vi "BiFuncHelp_MatrixMult.vi"(9 "B":T1, 10 "A":T1, 11 "Variant":variant) -> (0 "Error":bool, 3 "Output":T1)   [LabVIEW 2019, in "Trajectory_Library.lvlib"]
uses:
  Trajectory_Library.lvlib
  <vilib>/Analysis/Matrix/Datatypes/RealMatrix.ctl
  <vilib>/Analysis/baseanly.llb/Real A x B.vi
  <vilib>/Analysis/NI_AALBase.lvlib
  <vilib>/Analysis/Matrix/NI_Matrix.lvlib
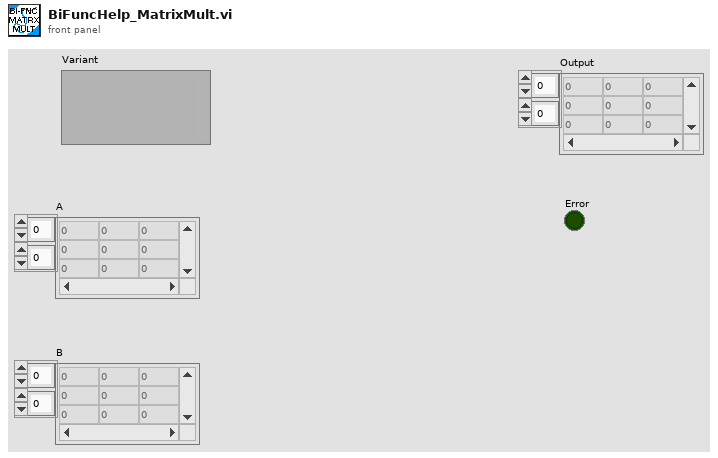
[diagram p1: front panel]
types:
  T1 = typedef "NI_Matrix.lvlib/RealMatrix.ctl" = dbl[][]
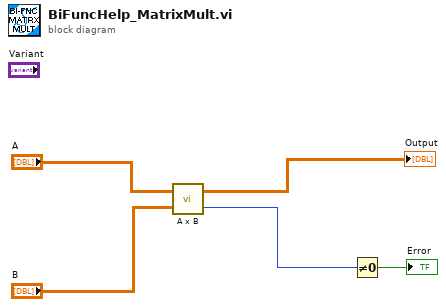
[diagram p0: block diagram]
diagram:
  n1 = call-poly <vilib>:"A x B.vi"("B"="B", "A"="A") -> ("error"=w2:i32, "A x B"=→"Output":T1)
  n2 = Not Equal To 0?(x=w2) -> (x != 0?=→"Error":bool)
